vi "BatchIterationGV.vi"(6 "SetMaxIteration":dbl, 8 "error in (no error)":errorcluster, 9 "SetIteration":dbl, 10 "GetOrSet":enum16{"Get", "Set"}(ring)) -> (0 "error out":errorcluster, 2 "Iteration":dbl, 4 "MaxIteration":dbl)   [LabVIEW 2016]
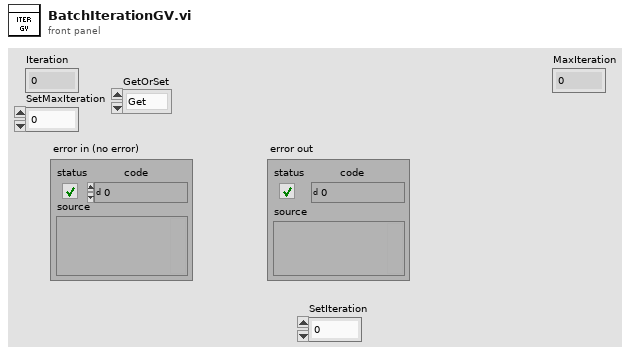
[diagram p1: front panel]
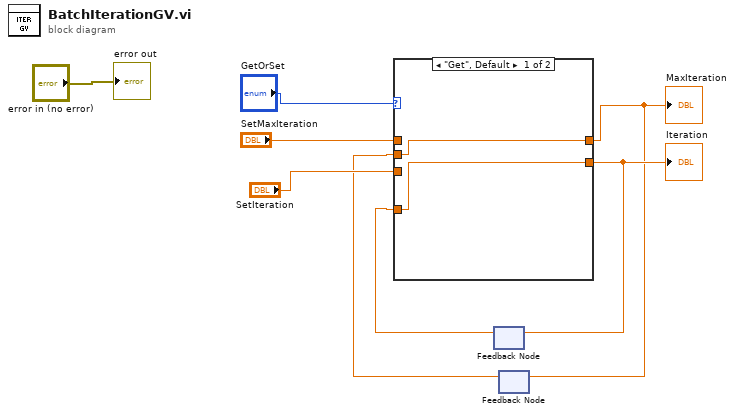
[diagram p0: block diagram]
diagram:
  n1 = feedback #1() -> (w5:dbl)  [unwired: 1 in]
  n2 = feedback #2() -> (w1:dbl)  [unwired: 1 in]
  n3 = case shown="\"Get\", Default" "GetOrSet" {
    tunnel: "SetIteration" -> [_ w12]
    tunnel: [w10 w12] -> w6
    tunnel: w5 -> [w10 _]
    tunnel: [w9 w11] -> w2
    tunnel: "SetMaxIteration" -> [_ w11]
    tunnel: w1 -> [w9 _]
    frame "Get", Default {
    }
    frame "Set" {
    }
  }
  "Iteration" <- w6
  "MaxIteration" <- w2
  n4 = feedback-in #1(w6) -> ()
  n5 = feedback-in #2(w2) -> ()
  "error out" <- "error in (no error)"
